vi "Read State Change Callback.vi"(11 "PersistantConnectionHandler in":refnum<class "PersistantConnectionHandler.lvclass">) -> (2 "State Change Callback":refnum<class "IConnectionStateChangeCallback.lvclass">, 3 "PersistantConnectionHandler out":refnum<class "PersistantConnectionHandler.lvclass">)   [LabVIEW 2020, in "PersitantConnectionHandler.lvlib" / "PersistantConnectionHandler.lvclass"]
uses:
  <vilib>/gpm_packages/@cs/Network-interface/Source/PersistantConnectionHandler/PersistantConnectionHandler/PersistantConnectionHandler.lvclass
  <vilib>/gpm_packages/@cs/Network-interface/Source/MessagingInterfaces/IConnectionStateChangeCallback/IConnectionStateChangeCallback.lvclass
  <vilib>/gpm_packages/@cs/Network-interface/Source/PersistantConnectionHandler/PersistantConnectionHandler/PersistantConnectionHandler.lvclass/PersistantConnectionHandler.ctl
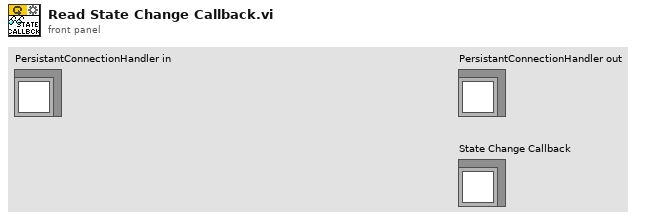
[diagram p1: front panel]
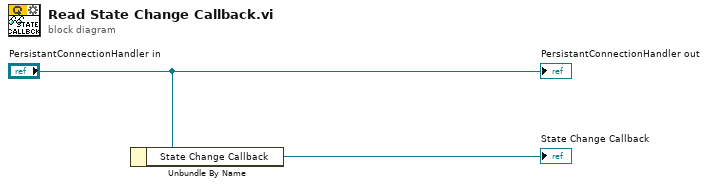
[diagram p0: block diagram]
diagram:
  n1 = Unbundle By Name("PersistantConnectionHandler in") -> ("State Change Callback"=→"State Change Callback":refnum<class "IConnectionStateChangeCallback.lvclass">)
  "PersistantConnectionHandler out" <- "PersistantConnectionHandler in"
